vi "Authenticate without Access Token.vi"(5 "Base URL":string, 6 "Body Parameters":T4[](array[typedef]), 7 "HTTP Method":T5, 8 "error in (no error)":errorcluster, 9 "Header Parameters":T4[](array[typedef]), 10 "URL Parameters":T4[](array[typedef]), 11 "OAuth Handle":T1={"Signature Method"=enum."HMAC-SHA1", "Version"="", "Client"={"Token"="", "Secret"=""}, "Access"={"Token"="", "Secret"=""}}) -> (0 "error out":errorcluster, 1 "Header Value":string, 2 "Header Parameter":string, 3 "Full URL":string, 4 "Body":string)   [LabVIEW 2011, in "i3-oauth.lvlib"]
doc: "<b>Note:</b> This function <b>DOES NOT</b> include the token secret and the token key for processing. The primary use of this VI is in the first stage of authentication before a request token / verification token / access token has been acquired. This VI is only needed if you are not using the Pin Access workflow provided and are instead implementing a custom OAUTH workflow (i.e. for embedded platforms, etc.)\n\nTakes parameters used for authenticated requests and creates the Auth HTTP Header Parameter and Value, performs x-www-form-urlencoding of Body Parameters, and adds url parameters to the base url to form the full url. \n\nAll parameters added to this VI (Body Parameters, URL Parameters, and Header Parameters) will be included in the OAUTH signature. Please read the API specification of the service being utilized to see which parameters should be included.\n\nExample:\nThe Twitter API v1.1 requires that when performing a POST that the status be added as a parameter to the body and included as part of the OAUTH signature. In this case the status is wired to the Body parameter of this function, it is used as part of the signature, and the x-www-form-urlencoded version of the body parameters are returned to send to Twitter. Alternatively the Twitter media multipart post specifies that the status and image are NOT added to the body so in this case the user will not include them as part of the signature and has to manually create the Post body"
uses:
  i3-oauth.lvlib
  Controls/Name-Value Pair.ctl
  Controls/HTTP Method.ctl
  Controls/OAuth Handle.ctl
  Controls/Signature Method.ctl
  Controls/Credentials.ctl
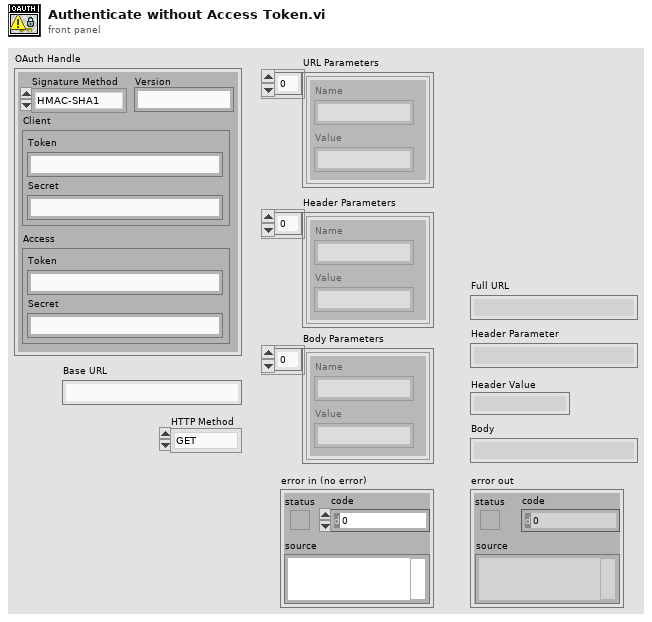
[diagram p1: front panel]
types:
  T1 = typedef "i3-oauth.lvlib/OAuth Handle.ctl" = cluster{"Signature Method":T2, "Version":string, "Client":T3, "Access":T3}
  T2 = typedef "i3-oauth.lvlib/Signature Method.ctl" = enum16{"HMAC-MD5", "HMAC-SHA1", "HMAC-SHA224", "HMAC-SHA256", "HMAC-SHA384", "HMAC-SHA512"}
  T3 = typedef "i3-oauth.lvlib/Credentials.ctl" = cluster{"Token":string, "Secret":string}
  T4 = typedef "i3-oauth.lvlib/Name-Value Pair.ctl" = cluster{"Name":string, "Value":string}
  T5 = typedef "i3-oauth.lvlib/HTTP Method.ctl" = enum16{"GET", "POST", "PUT", "DELETE"}
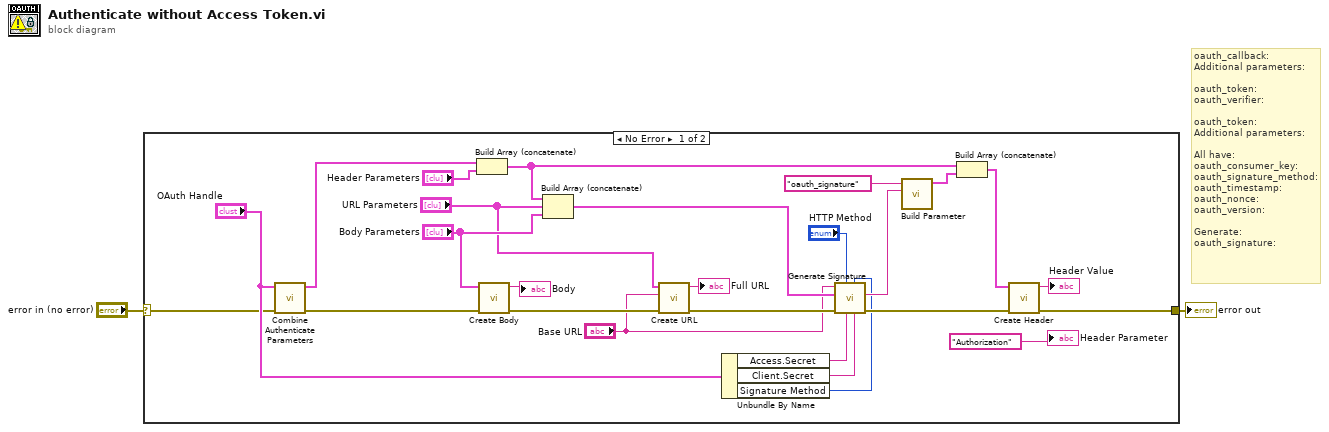
[diagram p0: block diagram]
diagram:
  # "oauth_callback:\nAdditional parameters:\n\noauth_token:\noauth_verifier:\n\noauth_token:\nAdditional parameters:\n\nAll have:\noauth_consumer_key:\noauth_signature_method:\noauth_timestamp:\noauth_nonce:\noauth_version:\n\nGenerate:\noauth_signature:"
  n1 = case shown="No Error" "error in (no error)" {
    selector: "error in (no error)" -> [w5 w29]
    tunnel: [w14 w29] -> w2
    frame No Error {
      n2 = call "Combine Authenticate Parameters.vi"("error in (no error)"=w5, "OAuth Credentials"="OAuth Handle") -> ("error out"=w6:errorcluster, "Authentication Parameters"=w19:T4[])  [unwired: 8 in]
      n3 = Build Array (concatenate)(w19, "Header Parameters") -> (w12:T4[])
      n4 = call "Create Body.vi"("error in (no error)"=w6, "Body Parameters"="Body Parameters") -> ("error out"=w23:errorcluster, "Body"=→"Body":string)  [unwired: 8 in]
      n5 = Build Array (concatenate)(w12, "URL Parameters", "Body Parameters") -> (w27:T4[])
      n6 = call "Create URL.vi"("error in (no error)"=w23, "Base URL"="Base URL", "URL Parameters"="URL Parameters") -> ("error out"=w28:errorcluster, "Full URL"=→"Full URL":string)  [unwired: 7 in]
      n7 = Unbundle By Name("OAuth Handle") -> ("Access.Secret"=w18:string, "Client.Secret"=w17:string, "Signature Method"=w13:T2)
      n8 = call "Generate Signature.vi"("consumer secret"=w17, "Signature Method"=w13, "access token secret"=w18, "HTTP Method"="HTTP Method", "error in (no error)"=w28, "Parameters"=w27, "Base URL"="Base URL") -> ("error out"=w25:errorcluster, "Signature"=w26:string)  [unwired: 3 in]
      n9 = call "Build Parameter.vi"("Value"=w26, "Key"="oauth_signature" ("key")) -> ("Parameter Array"=w9:T4[])  [unwired: 9 in]
      n10 = Build Array (concatenate)(w12, w9) -> (w11:T4[])
      n11 = call "Create Header.vi"("error in (no error)"=w25, "Header Parameters"=w11) -> ("error out"=w14:errorcluster, "Header"=→"Header Value":string)  [unwired: 8 in]
      "Header Parameter" <- "Authorization"
    }
    frame Error {
    }
  }
  "error out" <- w2
